vi "SubVI_Remove_Outliers.vi"(6 "Type":string="Both", 7 "Go Epochs":dbl[][](array[numeric]), 8 "error in (no error)":errorcluster, 9 "Proportion to delete":dbl, 10 "Rest Epochs":dbl[][](array[numeric]), 11 "Number of Trials":i32) -> (0 "error out":errorcluster, 1 "Rest Epochs":dbl[][](array[numeric]), 3 "Number of Trials":i32, 4 "Go Epochs":dbl[][](array[numeric]))   [LabVIEW 2020]
uses:
  <vilib>/Analysis/baseanly.llb/Mean (DBL).vi
  47a8b5ee-5992-4717-b8c2-1857c61fd609.vi
  b886193d-a7da-47ae-9726-84b609ffbc70.vi
  e91dfec7-f110-456b-bb68-98937f32c112.vi
  4428cf18-ebe8-4d0b-9418-2cdd673125c8.vi
  9453b5ee-2ccb-463d-903c-20b0ae4e3f16.vi
  6ef0763f-8b25-4be3-9027-8be35e33fe72.vi
  d7ffda31-33df-455c-8435-2436aa6314cb.vi
  e5e86f75-e4f1-46a5-afa4-0a2ec0139b83.vi
  12b11c3b-bfc6-4381-ae92-d1e4aa1180ee.vi
  <vilib>/Array/Sort 2D Array - Pop Stack.vi
  <vilib>/Array/Sort 2D Array - Push Stack.vi
  47a8b5ee-5992-4717-b8c2-1857c61fd609.vi/269d4b3b-47f5-49e3-8884-44851e4dd9d5.vi
  47a8b5ee-5992-4717-b8c2-1857c61fd609.vi/6d99389c-673d-4efb-bf33-19b32bcf4cf8.vi
  b886193d-a7da-47ae-9726-84b609ffbc70.vi/269d4b3b-47f5-49e3-8884-44851e4dd9d5.vi
  b886193d-a7da-47ae-9726-84b609ffbc70.vi/6d99389c-673d-4efb-bf33-19b32bcf4cf8.vi
  e91dfec7-f110-456b-bb68-98937f32c112.vi/269d4b3b-47f5-49e3-8884-44851e4dd9d5.vi
  e91dfec7-f110-456b-bb68-98937f32c112.vi/6d99389c-673d-4efb-bf33-19b32bcf4cf8.vi
  4428cf18-ebe8-4d0b-9418-2cdd673125c8.vi/269d4b3b-47f5-49e3-8884-44851e4dd9d5.vi
  4428cf18-ebe8-4d0b-9418-2cdd673125c8.vi/6d99389c-673d-4efb-bf33-19b32bcf4cf8.vi
  9453b5ee-2ccb-463d-903c-20b0ae4e3f16.vi/269d4b3b-47f5-49e3-8884-44851e4dd9d5.vi
  9453b5ee-2ccb-463d-903c-20b0ae4e3f16.vi/6d99389c-673d-4efb-bf33-19b32bcf4cf8.vi
  6ef0763f-8b25-4be3-9027-8be35e33fe72.vi/269d4b3b-47f5-49e3-8884-44851e4dd9d5.vi
  6ef0763f-8b25-4be3-9027-8be35e33fe72.vi/6d99389c-673d-4efb-bf33-19b32bcf4cf8.vi
  d7ffda31-33df-455c-8435-2436aa6314cb.vi/269d4b3b-47f5-49e3-8884-44851e4dd9d5.vi
  d7ffda31-33df-455c-8435-2436aa6314cb.vi/6d99389c-673d-4efb-bf33-19b32bcf4cf8.vi
  e5e86f75-e4f1-46a5-afa4-0a2ec0139b83.vi/269d4b3b-47f5-49e3-8884-44851e4dd9d5.vi
  e5e86f75-e4f1-46a5-afa4-0a2ec0139b83.vi/6d99389c-673d-4efb-bf33-19b32bcf4cf8.vi
  12b11c3b-bfc6-4381-ae92-d1e4aa1180ee.vi/269d4b3b-47f5-49e3-8884-44851e4dd9d5.vi
  12b11c3b-bfc6-4381-ae92-d1e4aa1180ee.vi/6d99389c-673d-4efb-bf33-19b32bcf4cf8.vi
  <vilib>/Analysis/NI_AALBase.lvlib
panel:
  out "Area mean (after) GO":dbl format="%e"
  out "Negative peak mean (after) GO":dbl format="%e"
  out "Slope mean (after) GO":dbl format="%e"
  out "Area mean (before) GO":dbl format="%e"
  out "Negative peak mean (before) GO":dbl format="%e"
  out "Slope mean (before) GO":dbl format="%e"
  out "Area mean (after) NO GO":dbl format="%e"
  out "Negative peak mean (after) NO GO":dbl format="%e"
  out "Slope mean (after) NO GO":dbl format="%e"
  out "Area mean (before) NO GO":dbl format="%e"
  out "Negative peak mean (before) NO GO":dbl format="%e"
  out "Slope mean (before) NO GO":dbl format="%e"
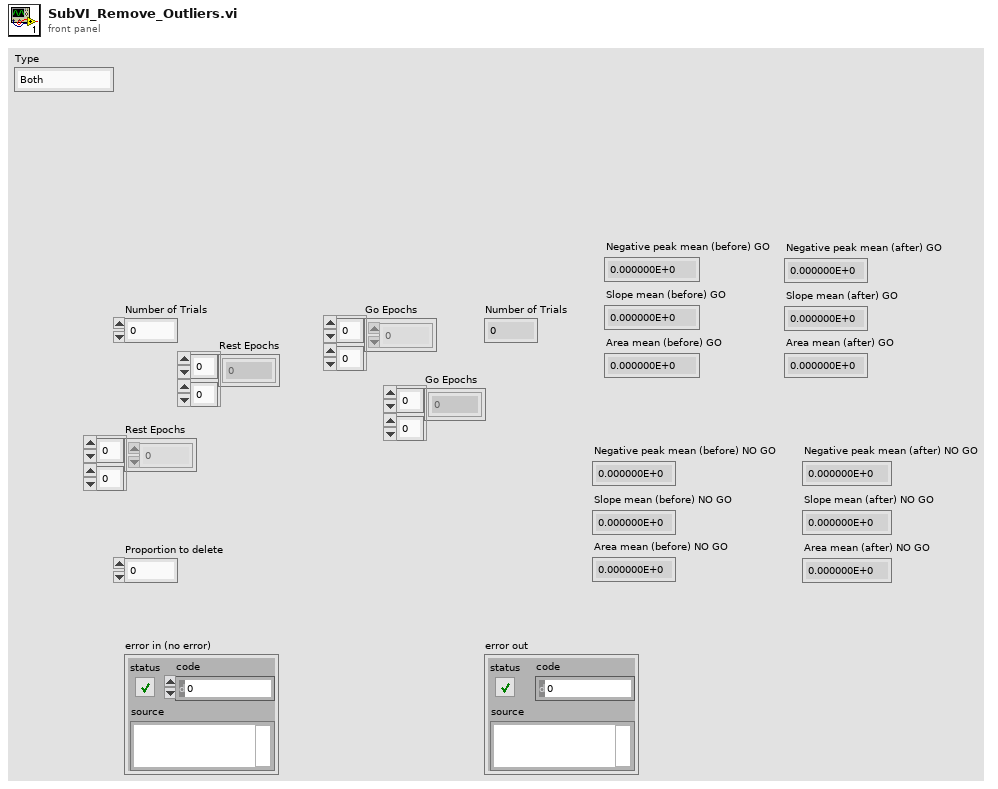
[diagram p1: front panel]
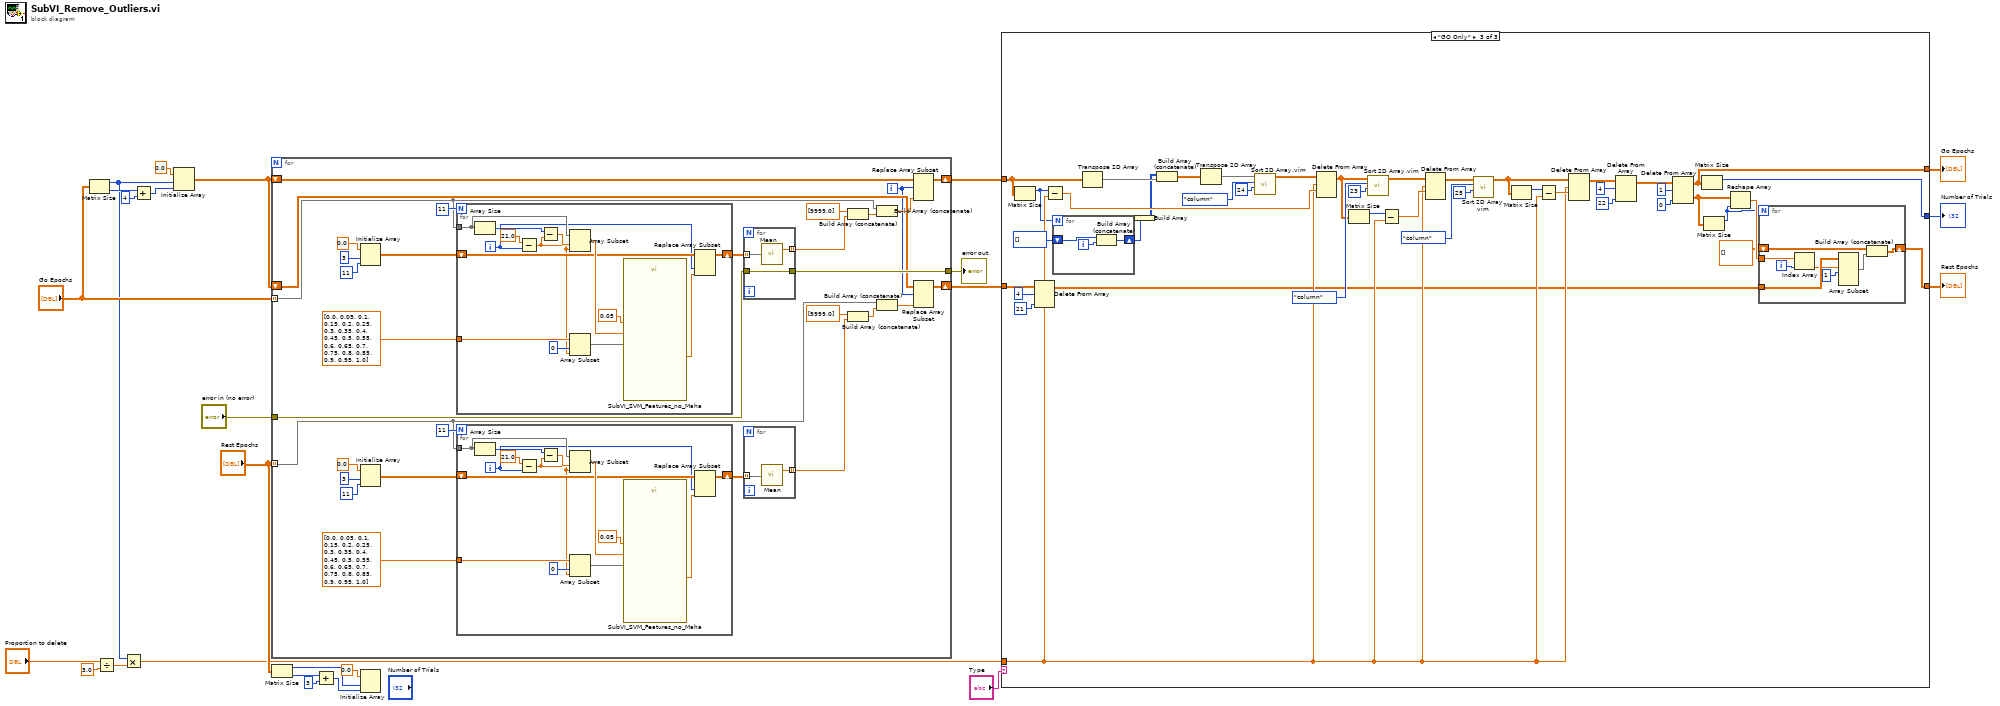
[diagram p0: block diagram]
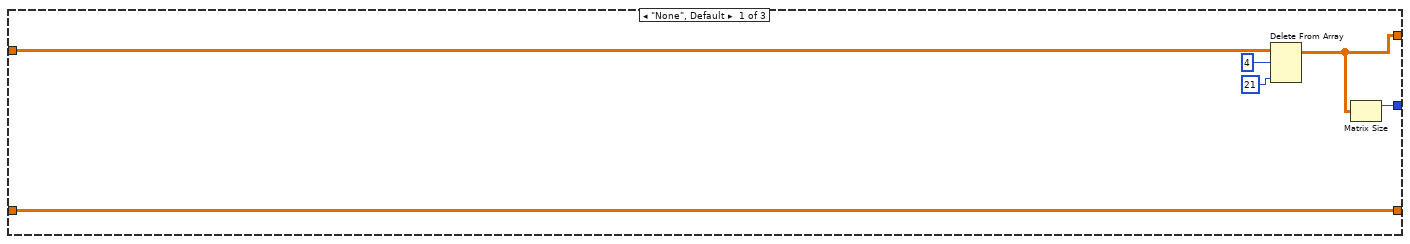
[diagram p2: hidden frame]
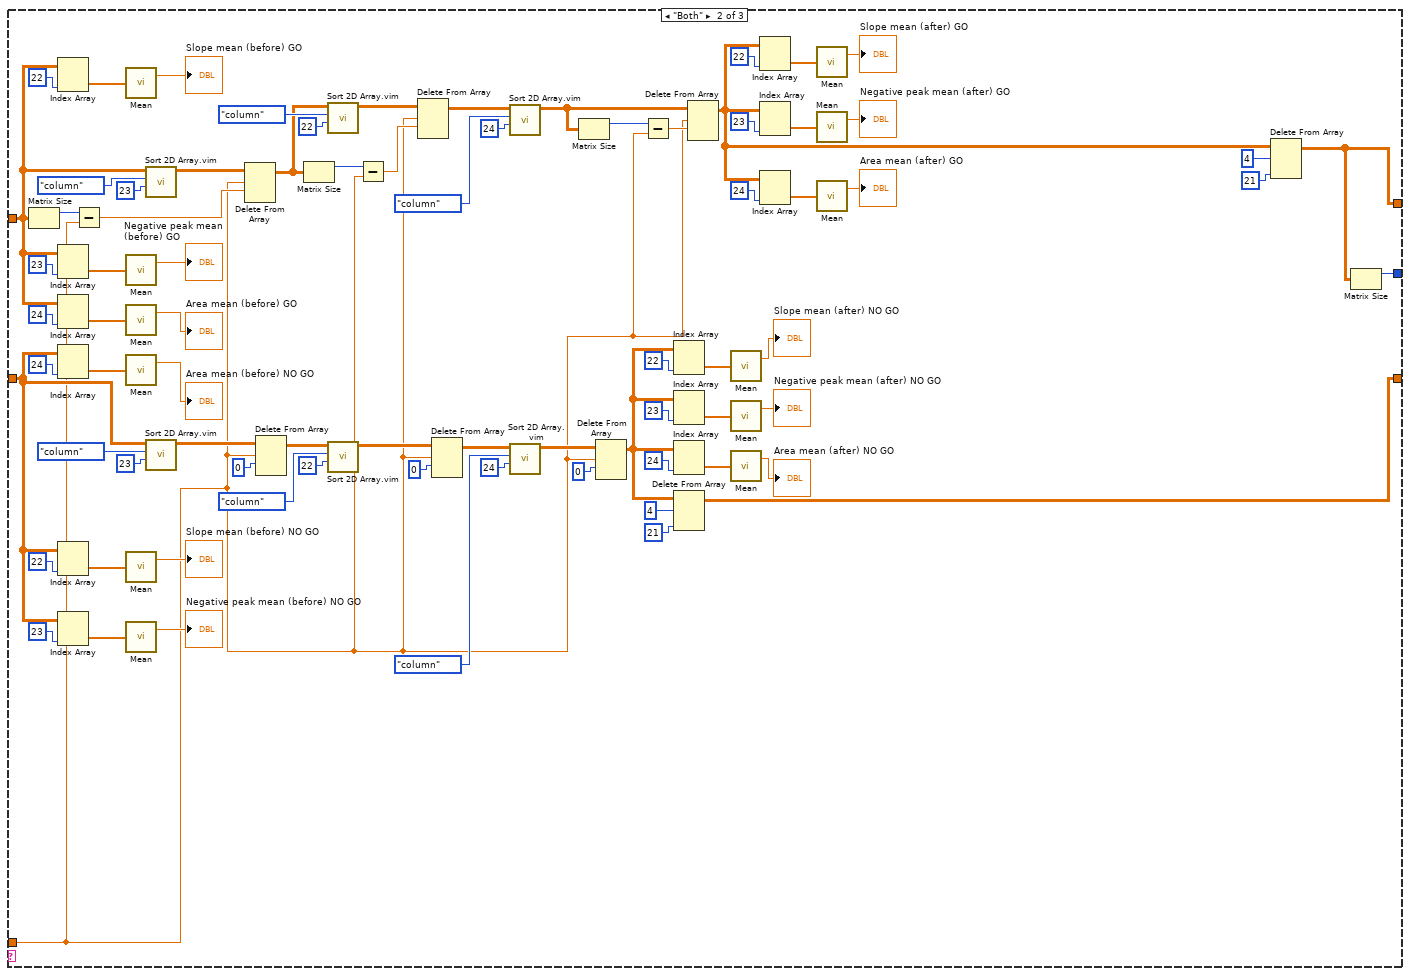
[diagram p3: hidden frame]
diagram:
  n1 = Matrix Size(0:"Go Epochs") -> (1:w7:i32, 2:w17:i32)
  n2 = Divide(x="Proportion to delete", y=3.0) -> (x/y=w3:dbl)
  n3 = Multiply(x=w7, y=w3) -> (x*y=w2:dbl)
  n4 = Add(x=w17, y=4) -> (x+y=w15:i32)
  n5 = Initialize Array(0.0 ("element"), w7, w15) -> (w9:dbl[][])
  n6 = for {
    tunnel: "Rest Epochs" -> [w28] mode=indexing
    tunnel: "Go Epochs" -> [w47] mode=indexing
    tunnel: "error in (no error)" -> [w49]
    tunnel: [w48] -> w23
    shift-right: [w44] -> w5
    shift-left: w9 -> [w46]
    shift-right: [w27] -> w6
    shift-left: w9 -> [w29]
    i -> [w26]
    n7 = Initialize Array(0.0 ("element"), 3 ("dimension size"), 11 ("dimension size")) -> (w51:dbl[][])
    n8 = Initialize Array(0.0 ("element"), 3 ("dimension size"), 11 ("dimension size")) -> (w35:dbl[][])
    n9 = for {
      N: 11 -> [_]
      tunnel: dbl[] [0.0, 0.05, 0.1, 0.15, 0.2, 0.25, 0.3, 0.35, 0.4, 0.45, 0.5, 0.55, 0.6, 0.65, 0.7, 0.75, 0.8, 0.85, 0.9, 0.95, 1.0] ("Sliding_window") -> [w84]
      tunnel: w47 -> [w87]
      shift-right: [w79] -> w50
      shift-left: w51 -> [w82]
      i -> [w81]
      n10 = Array Size(array=w87) -> (size(s)=w86:i32)
      n11 = Subtract(x=21.0, y=w81) -> (x-y=w76:dbl)
      n12 = Subtract(x=w86, y=w76) -> (x-y=w78:dbl)
      n13 = Array Subset(array=w87, index=w78, length=w76) -> (w85:dbl[])
      n14 = Array Subset(array=w84, index=0, length=w76) -> (w83:dbl[])
      n15 = call "SubVI_SVM_Features_no_Maha.vi"("dt"=0.05, "window_time"=w83, "Sliding_window"=w85) -> ("Features_array"=w80:dbl[])  [unwired: 5 in, 3 out]
      n16 = Replace Array Subset(array=w82, new element=w80, index (col)=w81) -> (w79:dbl[][])  [unwired: 1 in]
    }
    n17 = for {
      N: 11 -> [_]
      tunnel: dbl[] [0.0, 0.05, 0.1, 0.15, 0.2, 0.25, 0.3, 0.35, 0.4, 0.45, 0.5, 0.55, 0.6, 0.65, 0.7, 0.75, 0.8, 0.85, 0.9, 0.95, 1.0] ("Sliding_window") -> [w67]
      tunnel: w28 -> [w70]
      shift-right: [w62] -> w34
      shift-left: w35 -> [w65]
      i -> [w64]
      n18 = Array Size(array=w70) -> (size(s)=w69:i32)
      n19 = Subtract(x=21.0, y=w64) -> (x-y=w59:dbl)
      n20 = Subtract(x=w69, y=w59) -> (x-y=w61:dbl)
      n21 = Array Subset(array=w70, index=w61, length=w59) -> (w68:dbl[])
      n22 = Array Subset(array=w67, index=0, length=w59) -> (w66:dbl[])
      n23 = call "SubVI_SVM_Features_no_Maha.vi"("dt"=0.05, "window_time"=w66, "Sliding_window"=w68) -> ("Features_array"=w63:dbl[])  [unwired: 5 in, 3 out]
      n24 = Replace Array Subset(array=w65, new element=w63, index (col)=w64) -> (w62:dbl[][])  [unwired: 1 in]
    }
    n25 = for {
      tunnel: w50 -> [w75] mode=indexing
      tunnel: [w74] -> w43 mode=indexing
      tunnel: w49 -> [w73]
      tunnel: [w73] -> w48
      n26 = call-poly <vilib>:"Mean.vi"("X"=w75) -> ("mean"=w74:dbl)  [unwired: 1 out]
    }
    n27 = for {
      tunnel: w34 -> [w58] mode=indexing
      tunnel: [w57] -> w32 mode=indexing
      n28 = call-poly <vilib>:"Mean.vi"("X"=w58) -> ("mean"=w57:dbl)  [unwired: 1 out]
    }
    n29 = Build Array (concatenate)(dbl[] [9999.0] ("array"), w43) -> (w41:dbl[])
    n30 = Build Array (concatenate)(dbl[] [9999.0] ("array"), w32) -> (w30:dbl[])
    n31 = Build Array (concatenate)(w47, w41) -> (w45:dbl[])
    n32 = Build Array (concatenate)(w28, w30) -> (w33:dbl[])
    n33 = Replace Array Subset(array=w46, new element=w45, index (row)=w26) -> (w44:dbl[][])  [unwired: 1 in]
    n34 = Replace Array Subset(array=w29, new element=w33, index (row)=w26) -> (w27:dbl[][])  [unwired: 1 in]
  }
  "error out" <- w23
  n35 = Matrix Size(0:"Rest Epochs") -> (1:w10:i32, 2:w11:i32)
  n36 = Add(x=w11, y=3) -> (x+y=w12:i32)
  n37 = Initialize Array(0.0 ("element"), w10, w12) -> ()  [unwired: 1 out]
  n38 = case shown="\"GO Only\"" "Type" {
    tunnel: [w92 w174 w216] -> w24
    tunnel: [w91 w173 w187] -> w19
    tunnel: [w90 w172 w183] -> w18
    tunnel: w6 -> [w90 w140 w188]
    tunnel: w5 -> [w93 w102 w179]
    tunnel: w2 -> [_ w96 w194]
    frame "None", Default {
      n39 = Delete From Array(array=w93, length=4, index (col)=21) -> (array with subset deleted=w91:dbl[][])  [unwired: 1 in, 1 out]
      n40 = Matrix Size(0:w91) -> (1:w92:i32)  [unwired: 1 out]
    }
    frame "Both" {
      n41 = Matrix Size(0:w102) -> (1:w145:i32)  [unwired: 1 out]
      n42 = Index Array(array=w102, index (col)=22 ("disabled index (col)")) -> (element=w117:dbl[])  [unwired: 1 in]
      n43 = Index Array(array=w102, index (col)=23 ("disabled index (col)")) -> (element=w116:dbl[])  [unwired: 1 in]
      n44 = Index Array(array=w102, index (col)=24 ("disabled index (col)")) -> (element=w115:dbl[])  [unwired: 1 in]
      n45 = Index Array(array=w140, index (col)=24 ("disabled index (col)")) -> (element=w134:dbl[])  [unwired: 1 in]
      n46 = Index Array(array=w140, index (col)=22 ("disabled index (col)")) -> (element=w136:dbl[])  [unwired: 1 in]
      n47 = Index Array(array=w140, index (col)=23 ("disabled index (col)")) -> (element=w135:dbl[])  [unwired: 1 in]
      n48 = Subtract(x=w145, y=w96) -> (x-y=w144:dbl)
      n49 = call-poly <vilib>:"Mean.vi"("X"=w117) -> ("mean"=→"Slope mean (before) GO":dbl)  [unwired: 1 out]
      n50 = call-poly <vilib>:"Mean.vi"("X"=w116) -> ("mean"=→"Negative peak mean (before) GO":dbl)  [unwired: 1 out]
      n51 = call-poly <vilib>:"Mean.vi"("X"=w115) -> ("mean"=→"Area mean (before) GO":dbl)  [unwired: 1 out]
      n52 = call-poly <vilib>:"Mean.vi"("X"=w134) -> ("mean"=→"Area mean (before) NO GO":dbl)  [unwired: 1 out]
      n53 = call-poly <vilib>:"Mean.vi"("X"=w136) -> ("mean"=→"Slope mean (before) NO GO":dbl)  [unwired: 1 out]
      n54 = call-poly <vilib>:"Mean.vi"("X"=w135) -> ("mean"=→"Negative peak mean (before) NO GO":dbl)  [unwired: 1 out]
      n55 = call "Sort 2D Array.vim"("index"=23, "dimension to index (column)"=enum16{"column", "row"}."column", "2D array"=w102) -> ("sorted 2D array"=w169:dbl[][])  [unwired: 7 in, 1 out]
      n56 = call "Sort 2D Array.vim"("index"=23, "dimension to index (column)"=enum16{"column", "row"}."column", "2D array"=w140) -> ("sorted 2D array"=w157:dbl[][])  [unwired: 7 in, 1 out]
      n57 = Delete From Array(array=w169, length=w96, index (row)=w144) -> (array with subset deleted=w147:dbl[][])  [unwired: 1 in, 1 out]
      n58 = Delete From Array(array=w157, length=w96, index (row)=0) -> (array with subset deleted=w154:dbl[][])  [unwired: 1 in, 1 out]
      n59 = Matrix Size(0:w147) -> (1:w146:i32)  [unwired: 1 out]
      n60 = call "Sort 2D Array.vim"("index"=22, "dimension to index (column)"=enum16{"column", "row"}."column", "2D array"=w147) -> ("sorted 2D array"=w163:dbl[][])  [unwired: 7 in, 1 out]
      n61 = call "Sort 2D Array.vim"("index"=22, "dimension to index (column)"=enum16{"column", "row"}."column", "2D array"=w154) -> ("sorted 2D array"=w150:dbl[][])  [unwired: 7 in, 1 out]
      n62 = Subtract(x=w146, y=w96) -> (x-y=w162:dbl)
      n63 = Delete From Array(array=w163, length=w96, index (row)=w162) -> (array with subset deleted=w164:dbl[][])  [unwired: 1 in, 1 out]
      n64 = Delete From Array(array=w150, length=w96, index (row)=0) -> (array with subset deleted=w151:dbl[][])  [unwired: 1 in, 1 out]
      n65 = call "Sort 2D Array.vim"("index"=24, "dimension to index (column)"=enum16{"column", "row"}."column", "2D array"=w164) -> ("sorted 2D array"=w100:dbl[][])  [unwired: 7 in, 1 out]
      n66 = call "Sort 2D Array.vim"("index"=24, "dimension to index (column)"=enum16{"column", "row"}."column", "2D array"=w151) -> ("sorted 2D array"=w141:dbl[][])  [unwired: 7 in, 1 out]
      n67 = Matrix Size(0:w100) -> (1:w99:i32)  [unwired: 1 out]
      n68 = Delete From Array(array=w141, length=w96, index (row)=0) -> (array with subset deleted=w121:dbl[][])  [unwired: 1 in, 1 out]
      n69 = Subtract(x=w99, y=w96) -> (x-y=w98:dbl)
      n70 = Index Array(array=w121, index (col)=22 ("disabled index (col)")) -> (element=w127:dbl[])  [unwired: 1 in]
      n71 = Index Array(array=w121, index (col)=23 ("disabled index (col)")) -> (element=w126:dbl[])  [unwired: 1 in]
      n72 = Index Array(array=w121, index (col)=24 ("disabled index (col)")) -> (element=w125:dbl[])  [unwired: 1 in]
      n73 = Delete From Array(array=w121, length=4, index (col)=21) -> (array with subset deleted=w172:dbl[][])  [unwired: 1 in, 1 out]
      n74 = Delete From Array(array=w100, length=w96, index (row)=w98) -> (array with subset deleted=w101:dbl[][])  [unwired: 1 in, 1 out]
      n75 = call-poly <vilib>:"Mean.vi"("X"=w127) -> ("mean"=→"Slope mean (after) NO GO":dbl)  [unwired: 1 out]
      n76 = call-poly <vilib>:"Mean.vi"("X"=w126) -> ("mean"=→"Negative peak mean (after) NO GO":dbl)  [unwired: 1 out]
      n77 = call-poly <vilib>:"Mean.vi"("X"=w125) -> ("mean"=→"Area mean (after) NO GO":dbl)  [unwired: 1 out]
      n78 = Index Array(array=w101, index (col)=22 ("disabled index (col)")) -> (element=w108:dbl[])  [unwired: 1 in]
      n79 = Index Array(array=w101, index (col)=23 ("disabled index (col)")) -> (element=w107:dbl[])  [unwired: 1 in]
      n80 = Index Array(array=w101, index (col)=24 ("disabled index (col)")) -> (element=w106:dbl[])  [unwired: 1 in]
      n81 = call-poly <vilib>:"Mean.vi"("X"=w108) -> ("mean"=→"Slope mean (after) GO":dbl)  [unwired: 1 out]
      n82 = call-poly <vilib>:"Mean.vi"("X"=w107) -> ("mean"=→"Negative peak mean (after) GO":dbl)  [unwired: 1 out]
      n83 = call-poly <vilib>:"Mean.vi"("X"=w106) -> ("mean"=→"Area mean (after) GO":dbl)  [unwired: 1 out]
      n84 = Delete From Array(array=w101, length=4, index (col)=21) -> (array with subset deleted=w173:dbl[][])  [unwired: 1 in, 1 out]
      n85 = Matrix Size(0:w173) -> (1:w174:i32)  [unwired: 1 out]
    }
    frame "GO Only" {
      n86 = Matrix Size(0:w179) -> (1:w193:i32)  [unwired: 1 out]
      n87 = Delete From Array(array=w188, length=4, index (col)=21) -> (array with subset deleted=w186:dbl[][])  [unwired: 1 in, 1 out]
      n88 = Subtract(x=w193, y=w194) -> (x-y=w199:dbl)
      n89 = for {
        N: w193 -> [_]
        shift-right: [w227] -> w178
        shift-left: i32[] [] -> [w225]
        i -> [w226]
        n90 = Build Array (concatenate)(w225, w226) -> (w227:i32[])
      }
      n91 = Transpose 2D Array(2D array=w179) -> (transposed array=w182:dbl[][])
      n92 = Build Array(w178) -> (w177:i32[][])
      n93 = Build Array (concatenate)(w177, w182) -> (w192:dbl[][])
      n94 = Transpose 2D Array(2D array=w192) -> (transposed array=w181:dbl[][])
      n95 = call "Sort 2D Array.vim"("index"=24, "dimension to index (column)"=enum16{"column", "row"}."column", "2D array"=w181) -> ("sorted 2D array"=w213:dbl[][])  [unwired: 7 in, 1 out]
      n96 = Delete From Array(array=w213, length=w194, index (row)=w199) -> (array with subset deleted=w201:dbl[][])  [unwired: 1 in, 1 out]
      n97 = Matrix Size(0:w201) -> (1:w200:i32)  [unwired: 1 out]
      n98 = call "Sort 2D Array.vim"("index"=23, "dimension to index (column)"=enum16{"column", "row"}."column", "2D array"=w201) -> ("sorted 2D array"=w207:dbl[][])  [unwired: 7 in, 1 out]
      n99 = Subtract(x=w200, y=w194) -> (x-y=w206:dbl)
      n100 = Delete From Array(array=w207, length=w194, index (row)=w206) -> (array with subset deleted=w208:dbl[][])  [unwired: 1 in, 1 out]
      n101 = call "Sort 2D Array.vim"("index"=25, "dimension to index (column)"=enum16{"column", "row"}."column", "2D array"=w208) -> ("sorted 2D array"=w197:dbl[][])  [unwired: 7 in, 1 out]
      n102 = Matrix Size(0:w197) -> (1:w196:i32)  [unwired: 1 out]
      n103 = Subtract(x=w196, y=w194) -> (x-y=w195:dbl)
      n104 = Delete From Array(array=w197, length=w194, index (row)=w195) -> (array with subset deleted=w198:dbl[][])  [unwired: 1 in, 1 out]
      n105 = Delete From Array(array=w198, length=4, index (col)=22) -> (array with subset deleted=w191:dbl[][])  [unwired: 1 in, 1 out]
      n106 = Delete From Array(array=w191, length=1, index (col)=0 ("disabled index (col)")) -> (deleted portion=w185:dbl[][], array with subset deleted=w187:dbl[][])  [unwired: 1 in]
      n107 = Matrix Size(0:w187) -> (1:w216:i32)  [unwired: 1 out]
      n108 = Matrix Size(0:w185) -> (1:w180:i32)  [unwired: 1 out]
      n109 = Reshape Array(w185, w180) -> (w184:dbl[])
      n110 = for {
        N: w180 -> [_]
        tunnel: w186 -> [w224]
        tunnel: w184 -> [w218]
        shift-right: [w222] -> w183
        shift-left: dbl[][] [] -> [w220]
        i -> [w219]
        n111 = Index Array(array=w218, index=w219) -> (element=w217:dbl)
        n112 = Array Subset(array=w224, index (row)=w217, length (row)=1 ("length")) -> (w221:dbl[][])  [unwired: 2 in]
        n113 = Build Array (concatenate)(w220, w221) -> (w222:dbl[][])
      }
    }
  }
  "Number of Trials" <- w24
  "Go Epochs" <- w19
  "Rest Epochs" <- w18
